vi "Notifier_Send_Cluster.vi"(8 "ErrorIn":errorcluster, 11 "ClusterIn":T1={"Admin"={"Lvl"=enum."Admin", "Pwd"=""}, "RTConfig"={"Arm"=FALSE, "Number"=0.0, "String"="GPIB0::2::INSTR"}, "SMS"={"Enbl?"=FALSE, "Addr"=[]}, "FPGA"={"Target"=enum."1", "Channel"=enum."1", "Ref1"=refnum, "Ref2"=refnum}, "Config"={"UsrCfg"={"Paths"={"CfgFile"=path "", "LogFolder"=path "", "LogFile"=path "", "NAS path"=path "", "ThreshFile"=path "", "RedunFolder"=path ""}, "SampleRate"=12500.0}, "FP_User"={"#NoiseSums"=1, "Max_df"=1, "AvgAvg"=FALSE, "#Avg"=1, "AutoCenter"=FALSE, "Inclin"={"Vmin"=0.0, "Vmax"=0.0, "Angle_min"=0.0, "Angle_max"=0.0, "Offset"=0.0, "Pos_Neg"=FALSE}, "1"={"Cal_"={"Fine"=0.000213623046875, "Coarse_"=4194303.0}, "Beac"={"Fine"=4194303.0, "Coarse_"=1.0}, "Scale"={"Step4"=10000.0, "Step5"=4194303.0, "Step6"=1.0, "Step7"=10000.0}, "Offset"=0.0, "Scale_Noise"=4194303.0, "Scale_Step1"=65535.0, "Scale_In_RT"=1.0, "ScaleMeas"=0.999969482421875, "FreqsToRemove"=[0, 1633], "Width"=[0, 1633], "ScaleMeasEnum"=enum."50", "FilterEnab"=enum."Step 1"}, "2"={"Cal_"={"Fine"=0.000213623046875, "Coarse_"=4194303.0}, "Beac"={"Fine"=0.000213623046875, "Coarse_"=4194303.0}, "Scale"={"Step4"=0.0, "Step5"=4194303.0, "Step6"=1.0, "Step7"=10000.0}, "Offset"=0.0, "Scale_Noise"=4194303.0, "Scale_Step1"=65535.0, "Scale_In_RT"=1.0, "ScaleMeas"=0.999969482421875, "FreqsToRemove"=[0, 1633], "Width"=[0, 1633], "ScaleMeasEnum"=enum."50", "FilterEnab"=enum."Step 1"}, "3"={"Cal_"={"Fine"=0.000213623046875, "Coarse_"=4194303.0}, "Beac"={"Fine"=0.000213623046875, "Coarse_"=4194303.0}, "Scale"={"Step4"=0.0, "Step5"=4194303.0, "Step6"=1.0, "Step7"=10000.0}, "Offset"=0.0, "Scale_Noise"=4194303.0, "Scale_Step1"=65535.0, "Scale_In_RT"=1.0, "ScaleMeas"=0.999969482421875, "FreqsToRemove"=[0, 1633], "Width"=[0, 1633], "ScaleMeasEnum"=enum."50", "FilterEnab"=enum."Step 1"}, "4"={"Cal_"={"Fine"=0.000213623046875, "Coarse_"=4194303.0}, "Beac"={"Fine"=0.000213623046875, "Coarse_"=4194303.0}, "Scale"={"Step4"=0.0, "Step5"=4194303.0, "Step6"=1.0, "Step7"=10000.0}, "Offset"=0.0, "Scale_Noise"=4194303.0, "Scale_Step1"=1.0, "Scale_In_RT"=10000.0, "ScaleMeas"=0.999969482421875, "FreqsToRemove"=[0, 1633], "Width"=[0, 1633], "ScaleMeasEnum"=enum."50", "FilterEnab"=enum."Step 1"}, "Target to Probe"=enum."4", "SNR_Thresh"=1.0, "Paths"={"CfgFile"=path "", "LogFolder"=path "", "LogFile"=path "", "NAS path"=path "", "ThreshFile"=path "", "RedunFolder"=path ""}, "Connex_Location"="", "SimulateFPGA"=FALSE}}, "Stat"={"SysState"=enum."Init", "TrackRate"=FALSE, "AutoCentr"=FALSE}, "Alarm"={"TC13"={"Enbl"=FALSE, "ErrsAndWarns"={0.0, 5.663716814159292, 7.168141592920354, 8.584070796460177}}, "AI1"={"Enbl"=FALSE, "ErrsAndWarns"={0.0, 5.663716814159292, 7.168141592920354, 8.584070796460177}}, "AI2"={"Enbl"=FALSE, "ErrsAndWarns"={0.0, 5.663716814159292, 7.168141592920354, 8.584070796460177}}, "AI3"={"Enbl"=FALSE, "ErrsAndWarns"={0.0, 5.663716814159292, 7.168141592920354, 8.584070796460177}}, "AI4"={"Enbl"=FALSE, "ErrsAndWarns"={0.0, 5.663716814159292, 7.168141592920354, 8.584070796460177}}, "AI5"={"Enbl"=FALSE, "ErrsAndWarns"={0.0, 5.663716814159292, 7.168141592920354, 8.584070796460177}}, "AI6"={"Enbl"=FALSE, "ErrsAndWarns"={0.0, 5.663716814159292, 7.168141592920354, 8.584070796460177}}, "AI16"={"Enbl"=FALSE, "ErrsAndWarns"={0.0, 5.663716814159292, 7.168141592920354, 8.584070796460177}}, "AI17"={"Enbl"=FALSE, "ErrsAndWarns"={0.0, 5.663716814159292, 7.168141592920354, 8.584070796460177}}, "AI18"={"Enbl"=FALSE, "ErrsAndWarns"={0.0, 5.663716814159292, 7.168141592920354, 8.584070796460177}}, "AI19"={"Enbl"=FALSE, "ErrsAndWarns"={0.0, 5.663716814159292, 7.168141592920354, 8.584070796460177}}, "TE1"={"Enbl"=FALSE, "ErrsAndWarns"={0.0, 5.663716814159292, 7.168141592920354, 8.584070796460177}}, "TE2"={"Enbl"=TRUE, "ErrsAndWarns"={0.0, 5.663716814159292, 7.168141592920354, 8.584070796460177}}, "TE3"={"Enbl"=FALSE, "ErrsAndWarns"={0.0, 5.663716814159292, 7.168141592920354, 8.584070796460177}}, "ADAM1"={"Enbl"=FALSE, "ErrsAndWarns"={0.0, 5.663716814159292, 7.168141592920354, 8.584070796460177}}, "ADAM2"={"Enbl"=FALSE, "ErrsAndWarns"={0.0, 5.663716814159292, 7.168141592920354, 8.584070796460177}}, "ADAM3"={"Enbl"=FALSE, "ErrsAndWarns"={0.0, 5.663716814159292, 7.168141592920354, 8.584070796460177}}, "ADAM4"={"Enbl"=FALSE, "ErrsAndWarns"={0.0, 5.663716814159292, 7.168141592920354, 8.584070796460177}}, "72CoBeacFreq"={"Enbl"=FALSE, "ErrsAndWarns"={0.0, 5.663716814159292, 7.168141592920354, 8.584070796460177}}, "72CoCalFreq"={"Enbl"=FALSE, "ErrsAndWarns"={0.0, 5.663716814159292, 7.168141592920354, 8.584070796460177}}, "72XBeacFreq"={"Enbl"=FALSE, "ErrsAndWarns"={0.0, 5.663716814159292, 7.168141592920354, 8.584070796460177}}, "72XCalFreq"={"Enbl"=FALSE, "ErrsAndWarns"={0.0, 5.663716814159292, 7.168141592920354, 8.584070796460177}}, "84CoBeacFreq"={"Enbl"=FALSE, "ErrsAndWarns"={0.0, 5.663716814159292, 7.168141592920354, 8.584070796460177}}, "84CoCalFreq"={"Enbl"=FALSE, "ErrsAndWarns"={0.0, 5.663716814159292, 7.168141592920354, 8.584070796460177}}, "84XBeacFreq"={"Enbl"=FALSE, "ErrsAndWarns"={0.0, 5.663716814159292, 7.168141592920354, 8.584070796460177}}, "84XCalFreq"={"Enbl"=FALSE, "ErrsAndWarns"={0.0, 5.663716814159292, 7.168141592920354, 8.584070796460177}}}} {"Alarm"."84XCalFreq"."ErrsAndWarns" scale=0.0..10.0; "Alarm"."84XBeacFreq"."ErrsAndWarns" scale=0.0..10.0; "Alarm"."84CoCalFreq"."ErrsAndWarns" scale=0.0..10.0; "Alarm"."84CoBeacFreq"."ErrsAndWarns" scale=0.0..10.0; "Alarm"."72XCalFreq"."ErrsAndWarns" scale=0.0..10.0; "Alarm"."72XBeacFreq"."ErrsAndWarns" scale=0.0..10.0; "Alarm"."72CoCalFreq"."ErrsAndWarns" scale=0.0..10.0; "Alarm"."72CoBeacFreq"."ErrsAndWarns" scale=0.0..10.0; "Alarm"."ADAM4"."ErrsAndWarns" scale=0.0..10.0; "Alarm"."ADAM3"."ErrsAndWarns" scale=0.0..10.0; "Alarm"."ADAM2"."ErrsAndWarns" scale=0.0..10.0; "Alarm"."ADAM1"."ErrsAndWarns" scale=0.0..10.0; "Alarm"."TE3"."ErrsAndWarns" scale=0.0..10.0; "Alarm"."TE2"."ErrsAndWarns" scale=0.0..10.0; "Alarm"."TE1"."ErrsAndWarns" scale=0.0..10.0; "Alarm"."AI19"."ErrsAndWarns" scale=0.0..10.0; "Alarm"."AI18"."ErrsAndWarns" scale=0.0..10.0; "Alarm"."AI17"."ErrsAndWarns" scale=0.0..10.0; "Alarm"."AI16"."ErrsAndWarns" scale=0.0..10.0; "Alarm"."AI6"."ErrsAndWarns" scale=0.0..10.0; "Alarm"."AI5"."ErrsAndWarns" scale=0.0..10.0; "Alarm"."AI4"."ErrsAndWarns" scale=0.0..10.0; "Alarm"."AI3"."ErrsAndWarns" scale=0.0..10.0; "Alarm"."AI2"."ErrsAndWarns" scale=0.0..10.0; "Alarm"."AI1"."ErrsAndWarns" scale=0.0..10.0; "Alarm"."TC13"."ErrsAndWarns" scale=0.0..10.0}) -> (0 "ErrorOut":errorcluster, 3 "ClusterOut":T1={"Admin"={"Lvl"=enum."Admin", "Pwd"=""}, "RTConfig"={"Arm"=FALSE, "Number"=0.0, "String"="GPIB0::2::INSTR"}, "SMS"={"Enbl?"=FALSE, "Addr"=[]}, "FPGA"={"Target"=enum."1", "Channel"=enum."1", "Ref1"=refnum, "Ref2"=refnum}, "Config"={"UsrCfg"={"Paths"={"CfgFile"=path "", "LogFolder"=path "", "LogFile"=path "", "NAS path"=path "", "ThreshFile"=path "", "RedunFolder"=path ""}, "SampleRate"=12500.0}, "FP_User"={"#NoiseSums"=1, "Max_df"=1, "AvgAvg"=FALSE, "#Avg"=1, "AutoCenter"=FALSE, "Inclin"={"Vmin"=0.0, "Vmax"=0.0, "Angle_min"=0.0, "Angle_max"=0.0, "Offset"=0.0, "Pos_Neg"=FALSE}, "1"={"Cal_"={"Fine"=0.000213623046875, "Coarse_"=4194303.0}, "Beac"={"Fine"=4194303.0, "Coarse_"=1.0}, "Scale"={"Step4"=10000.0, "Step5"=4194303.0, "Step6"=1.0, "Step7"=10000.0}, "Offset"=0.0, "Scale_Noise"=4194303.0, "Scale_Step1"=65535.0, "Scale_In_RT"=1.0, "ScaleMeas"=0.999969482421875, "FreqsToRemove"=[0, 1633], "Width"=[0, 1633], "ScaleMeasEnum"=enum."50", "FilterEnab"=enum."Step 1"}, "2"={"Cal_"={"Fine"=0.000213623046875, "Coarse_"=4194303.0}, "Beac"={"Fine"=0.000213623046875, "Coarse_"=4194303.0}, "Scale"={"Step4"=0.0, "Step5"=4194303.0, "Step6"=1.0, "Step7"=10000.0}, "Offset"=0.0, "Scale_Noise"=4194303.0, "Scale_Step1"=65535.0, "Scale_In_RT"=1.0, "ScaleMeas"=0.999969482421875, "FreqsToRemove"=[0, 1633], "Width"=[0, 1633], "ScaleMeasEnum"=enum."50", "FilterEnab"=enum."Step 1"}, "3"={"Cal_"={"Fine"=0.000213623046875, "Coarse_"=4194303.0}, "Beac"={"Fine"=0.000213623046875, "Coarse_"=4194303.0}, "Scale"={"Step4"=0.0, "Step5"=4194303.0, "Step6"=1.0, "Step7"=10000.0}, "Offset"=0.0, "Scale_Noise"=4194303.0, "Scale_Step1"=65535.0, "Scale_In_RT"=1.0, "ScaleMeas"=0.999969482421875, "FreqsToRemove"=[0, 1633], "Width"=[0, 1633], "ScaleMeasEnum"=enum."50", "FilterEnab"=enum."Step 1"}, "4"={"Cal_"={"Fine"=0.000213623046875, "Coarse_"=4194303.0}, "Beac"={"Fine"=0.000213623046875, "Coarse_"=4194303.0}, "Scale"={"Step4"=0.0, "Step5"=4194303.0, "Step6"=1.0, "Step7"=10000.0}, "Offset"=0.0, "Scale_Noise"=4194303.0, "Scale_Step1"=1.0, "Scale_In_RT"=10000.0, "ScaleMeas"=0.999969482421875, "FreqsToRemove"=[0, 1633], "Width"=[0, 1633], "ScaleMeasEnum"=enum."50", "FilterEnab"=enum."Step 1"}, "Target to Probe"=enum."4", "SNR_Thresh"=1.0, "Paths"={"CfgFile"=path "", "LogFolder"=path "", "LogFile"=path "", "NAS path"=path "", "ThreshFile"=path "", "RedunFolder"=path ""}, "Connex_Location"="", "SimulateFPGA"=FALSE}}, "Stat"={"SysState"=enum."Init", "TrackRate"=FALSE, "AutoCentr"=FALSE}, "Alarm"={"TC13"={"Enbl"=FALSE, "ErrsAndWarns"={0.0, 5.663716814159292, 7.168141592920354, 8.584070796460177}}, "AI1"={"Enbl"=FALSE, "ErrsAndWarns"={0.0, 5.663716814159292, 7.168141592920354, 8.584070796460177}}, "AI2"={"Enbl"=FALSE, "ErrsAndWarns"={0.0, 5.663716814159292, 7.168141592920354, 8.584070796460177}}, "AI3"={"Enbl"=FALSE, "ErrsAndWarns"={0.0, 5.663716814159292, 7.168141592920354, 8.584070796460177}}, "AI4"={"Enbl"=FALSE, "ErrsAndWarns"={0.0, 5.663716814159292, 7.168141592920354, 8.584070796460177}}, "AI5"={"Enbl"=FALSE, "ErrsAndWarns"={0.0, 5.663716814159292, 7.168141592920354, 8.584070796460177}}, "AI6"={"Enbl"=FALSE, "ErrsAndWarns"={0.0, 5.663716814159292, 7.168141592920354, 8.584070796460177}}, "AI16"={"Enbl"=FALSE, "ErrsAndWarns"={0.0, 5.663716814159292, 7.168141592920354, 8.584070796460177}}, "AI17"={"Enbl"=FALSE, "ErrsAndWarns"={0.0, 5.663716814159292, 7.168141592920354, 8.584070796460177}}, "AI18"={"Enbl"=FALSE, "ErrsAndWarns"={0.0, 5.663716814159292, 7.168141592920354, 8.584070796460177}}, "AI19"={"Enbl"=FALSE, "ErrsAndWarns"={0.0, 5.663716814159292, 7.168141592920354, 8.584070796460177}}, "TE1"={"Enbl"=FALSE, "ErrsAndWarns"={0.0, 5.663716814159292, 7.168141592920354, 8.584070796460177}}, "TE2"={"Enbl"=TRUE, "ErrsAndWarns"={0.0, 5.663716814159292, 7.168141592920354, 8.584070796460177}}, "TE3"={"Enbl"=FALSE, "ErrsAndWarns"={0.0, 5.663716814159292, 7.168141592920354, 8.584070796460177}}, "ADAM1"={"Enbl"=FALSE, "ErrsAndWarns"={0.0, 5.663716814159292, 7.168141592920354, 8.584070796460177}}, "ADAM2"={"Enbl"=FALSE, "ErrsAndWarns"={0.0, 5.663716814159292, 7.168141592920354, 8.584070796460177}}, "ADAM3"={"Enbl"=FALSE, "ErrsAndWarns"={0.0, 5.663716814159292, 7.168141592920354, 8.584070796460177}}, "ADAM4"={"Enbl"=FALSE, "ErrsAndWarns"={0.0, 5.663716814159292, 7.168141592920354, 8.584070796460177}}, "72CoBeacFreq"={"Enbl"=FALSE, "ErrsAndWarns"={0.0, 5.663716814159292, 7.168141592920354, 8.584070796460177}}, "72CoCalFreq"={"Enbl"=FALSE, "ErrsAndWarns"={0.0, 5.663716814159292, 7.168141592920354, 8.584070796460177}}, "72XBeacFreq"={"Enbl"=FALSE, "ErrsAndWarns"={0.0, 5.663716814159292, 7.168141592920354, 8.584070796460177}}, "72XCalFreq"={"Enbl"=FALSE, "ErrsAndWarns"={0.0, 5.663716814159292, 7.168141592920354, 8.584070796460177}}, "84CoBeacFreq"={"Enbl"=FALSE, "ErrsAndWarns"={0.0, 5.663716814159292, 7.168141592920354, 8.584070796460177}}, "84CoCalFreq"={"Enbl"=FALSE, "ErrsAndWarns"={0.0, 5.663716814159292, 7.168141592920354, 8.584070796460177}}, "84XBeacFreq"={"Enbl"=FALSE, "ErrsAndWarns"={0.0, 5.663716814159292, 7.168141592920354, 8.584070796460177}}, "84XCalFreq"={"Enbl"=FALSE, "ErrsAndWarns"={0.0, 5.663716814159292, 7.168141592920354, 8.584070796460177}}}} {"Alarm"."84XCalFreq"."ErrsAndWarns" scale=0.0..10.0; "Alarm"."84XBeacFreq"."ErrsAndWarns" scale=0.0..10.0; "Alarm"."84CoCalFreq"."ErrsAndWarns" scale=0.0..10.0; "Alarm"."84CoBeacFreq"."ErrsAndWarns" scale=0.0..10.0; "Alarm"."72XCalFreq"."ErrsAndWarns" scale=0.0..10.0; "Alarm"."72XBeacFreq"."ErrsAndWarns" scale=0.0..10.0; "Alarm"."72CoCalFreq"."ErrsAndWarns" scale=0.0..10.0; "Alarm"."72CoBeacFreq"."ErrsAndWarns" scale=0.0..10.0; "Alarm"."ADAM4"."ErrsAndWarns" scale=0.0..10.0; "Alarm"."ADAM3"."ErrsAndWarns" scale=0.0..10.0; "Alarm"."ADAM2"."ErrsAndWarns" scale=0.0..10.0; "Alarm"."ADAM1"."ErrsAndWarns" scale=0.0..10.0; "Alarm"."TE3"."ErrsAndWarns" scale=0.0..10.0; "Alarm"."TE2"."ErrsAndWarns" scale=0.0..10.0; "Alarm"."TE1"."ErrsAndWarns" scale=0.0..10.0; "Alarm"."AI19"."ErrsAndWarns" scale=0.0..10.0; "Alarm"."AI18"."ErrsAndWarns" scale=0.0..10.0; "Alarm"."AI17"."ErrsAndWarns" scale=0.0..10.0; "Alarm"."AI16"."ErrsAndWarns" scale=0.0..10.0; "Alarm"."AI6"."ErrsAndWarns" scale=0.0..10.0; "Alarm"."AI5"."ErrsAndWarns" scale=0.0..10.0; "Alarm"."AI4"."ErrsAndWarns" scale=0.0..10.0; "Alarm"."AI3"."ErrsAndWarns" scale=0.0..10.0; "Alarm"."AI2"."ErrsAndWarns" scale=0.0..10.0; "Alarm"."AI1"."ErrsAndWarns" scale=0.0..10.0; "Alarm"."TC13"."ErrsAndWarns" scale=0.0..10.0})   [LabVIEW 2018]
doc: "Bundle the latest MasterCluster (<B>ClusterIn</B>) into the existing notifier member of the MasterCluster and send it to the loops that need this updated cluster, such as the Hardware Loop. In general, this is used to pass updated information to the Hardware Loop whenever a state change has occured in the Main (Consumer) Loop.\n\n<B>ClusterOut</B> is the same as <B>ClusterIn</B>.\n\nAlso See Notifier_Send.vi\n\nA notifier is useful for a one-to-one or one-to-many flow from one loop to others.\n\nCopyright © 2011 Epimedia, Inc. All Rights Reserved.\n\nThe Epimedia Application Library is Copyright © 2009-2011 Epimedia, Inc. \nAll Rights Reserved. Used under license."
uses:
  Controls/PathsCluster.ctl
  Controls/UserLevelEnum.ctl
  Controls/MasterCluster.ctl
  Controls/SystemStatusCluster.ctl
  Controls/SystemStateEnum.ctl
  Controls/Clusts/AdminCluster.ctl
  Controls/RT_Config.ctl
  Controls/SMSDataCluster.ctl
  Controls/Enums/TargetNumber.ctl
  Controls/Clusts/FPGA_Config_Clust.ctl
  Controls/Clusts/UserConfig.ctl
  Controls/Clusts/FreqShift.ctl
  Controls/Clusts/FPGA_Scale.ctl
  Controls/Enums/ScaleMeasure.ctl
  Controls/RadioButtons/FilterEnableRadio.ctl
  Controls/Clusts/FP_UserTargetConfig.ctl
  Controls/Clusts/Inclinometer_User_Cfg.ctl
  Controls/Clusts/FrontPanel_UserConfig.ctl
  Controls/Clusts/Config_Clust.ctl
  Controls/Clusts/AlarmThresh_OneChan.ctl
  Controls/Clusts/AlarmSettingsClust.ctl
panel:
  # "Copyright © 2011 Epimedia, Inc. All Rights Reserved.\n\nThe Epimedia Application Library is Copyright © 2009-2011 Epimedia, Inc. \nAll Rights Reserved. Used under license."
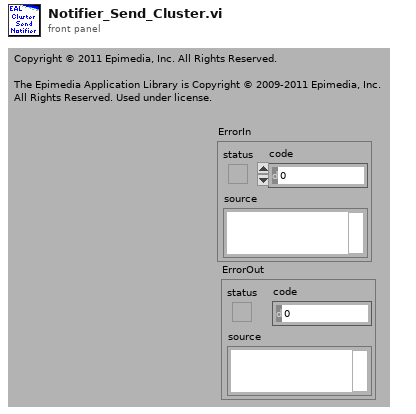
[diagram p1: front panel]
types:
  T1 = typedef "MasterCluster.ctl" = cluster{"Admin":T2, "RTConfig":T4, "SMS":T5, "FPGA":T6, "Config":T8, "Stat":T18, "Alarm":T20}
  T2 = typedef "AdminCluster.ctl" = cluster{"Lvl":T3, "Pwd":string}
  T3 = typedef "UserLevelEnum.ctl" = enum16{"Admin", "Operator"}
  T4 = typedef "RT_Config.ctl" = cluster{"Arm":bool, "Number":dbl, "String":string}
  T5 = typedef "SMSDataCluster.ctl" = cluster{"Enbl?":bool, "Addr":string[]}
  T6 = typedef "FPGA_Config_Clust.ctl" = cluster{"Target":T7, "Channel":T7, "Ref1":refnum<k20>, "Ref2":refnum<k20>}
  T7 = typedef "TargetNumber.ctl" = enum16{"1", "2", "3", "4"}
  T8 = typedef "Config_Clust.ctl" = cluster{"UsrCfg":T9, "FP_User":T11}
  T9 = typedef "UserConfig.ctl" = cluster{"Paths":T10, "SampleRate":dbl}
  T10 = typedef "PathsCluster.ctl" = cluster{"CfgFile":path, "LogFolder":path, "LogFile":path, "NAS path":path, "ThreshFile":path, "RedunFolder":path}
  T11 = typedef "FrontPanel_UserConfig.ctl" = cluster{"#NoiseSums":u32, "Max_df":u32, "AvgAvg":bool, "#Avg":u16, "AutoCenter":bool, "Inclin":T12, "1":T13, "2":T13, "3":T13, "4":T13, "Target to Probe":T7, "SNR_Thresh":dbl, "Paths":T10, "Connex_Location":string, "SimulateFPGA":bool}
  T12 = typedef "Inclinometer_User_Cfg.ctl" = cluster{"Vmin":dbl, "Vmax":dbl, "Angle_min":dbl, "Angle_max":dbl, "Offset":dbl, "Pos_Neg":bool}
  T13 = typedef "FP_UserTargetConfig.ctl" = cluster{"Cal_":T14, "Beac":T14, "Scale":T15, "Offset":fxp<+/-,16,16>, "Scale_Noise":fxp<+/-,30,30>, "Scale_Step1":fxp<+/-,17,17>, "Scale_In_RT":ext, "ScaleMeas":fxp<+/-,16,1>, "FreqsToRemove":i32[], "Width":i32[], "ScaleMeasEnum":T16, "FilterEnab":T17}
  T14 = typedef "FreqShift.ctl" = cluster{"Fine":dbl, "Coarse_":dbl}
  T15 = typedef "FPGA_Scale.ctl" = cluster{"Step4":fxp<+/-,23,23>, "Step5":fxp<+/-,23,23>, "Step6":fxp<+/-,23,23>, "Step7":fxp<+/-,23,23>}
  T16 = typedef "ScaleMeasure.ctl" = enum16{"1", "10", "50", "42"}
  T17 = typedef "FilterEnableRadio.ctl" = enum32{"None", "Step 1", "Frequency Shift", "Step 4", "Step 5", "Step 6", "Step 7"}
  T18 = typedef "SystemStatusCluster.ctl" = cluster{"SysState":T19, "TrackRate":bool, "AutoCentr":bool}
  T19 = typedef "SystemStateEnum.ctl" = enum16{"Init", "Idle", "Running", "System Fault", "System Error", "Exit"}
  T20 = typedef "AlarmSettingsClust.ctl" = cluster{"TC13":T21, "AI1":T21, "AI2":T21, "AI3":T21, "AI4":T21, "AI5":T21, "AI6":T21, "AI16":T21, "AI17":T21, "AI18":T21, "AI19":T21, "TE1":T21, "TE2":T21, "TE3":T21, "ADAM1":T21, "ADAM2":T21, "ADAM3":T21, "ADAM4":T21, "72CoBeacFreq":T21, "72CoCalFreq":T21, "72XBeacFreq":T21, "72XCalFreq":T21, "84CoBeacFreq":T21, "84CoCalFreq":T21, "84XBeacFreq":T21, "84XCalFreq":T21}
  T21 = typedef "AlarmThresh_OneChan.ctl" = cluster{"Enbl":bool, "ErrsAndWarns":cluster{dbl, dbl, dbl, dbl}}
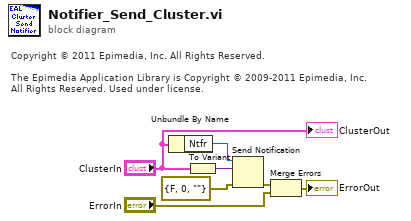
[diagram p0: block diagram]
diagram:
  # "Copyright © 2011 Epimedia, Inc. All Rights Reserved.\n\nThe Epimedia Application Library is Copyright © 2009-2011 Epimedia, Inc. \nAll Rights Reserved. Used under license."
  n1 = Unbundle By Name("ClusterIn") -> ("Ntfr"=w5:refnum<notifier>)
  n2 = To Variant(anything="ClusterIn") -> (Variant=w7:variant)
  n3 = Send Notification(notification=w7, notifier=w5, error in (no error)=errorcluster {"status"=FALSE, "code"=0, "source"=""}) -> (error out=w4:errorcluster)  [unwired: 1 out]
  n4 = Merge Errors(w4, "ErrorIn") -> (→"ErrorOut":errorcluster)
  "ClusterOut" <- "ClusterIn"
